vi "1 channel 1 sample (temperature measurement).vi"() -> ()   [LabVIEW 2020]
panel:
  out "deg":dbl(knob) scale=-100.0..100.0
  out "degree c":dbl
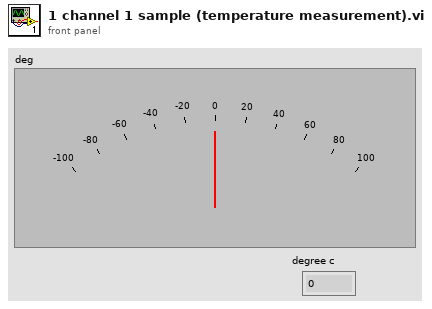
[diagram p1: front panel]
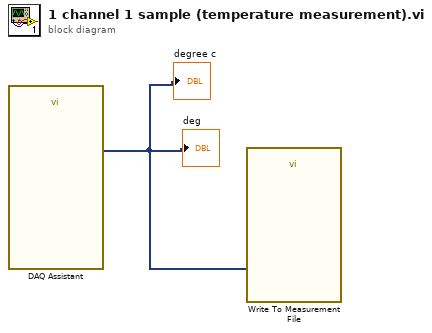
[diagram p0: block diagram]
diagram:
  n1 = call "DAQ Assistant"() -> ("data"=w1:dynamicdata)  [unwired: 17 in, 2 out]
  "degree c" <- w1
  "deg" <- w1
  n2 = call "Write To Measurement File"("Signals"=w1) -> ()  [unwired: 16 in, 3 out]
